vi "ThreePts_RotationMatrix.vi"(2 "Circumcenter":dbl[](array[numeric]), 3 "V 2":dbl[](array[numeric]), 4 "V 1":dbl[](array[numeric])) -> (0 "Circumcenter":dbl[](array[numeric]), 1 "Rotation Matrix ( Local to Global )":dbl[][](array[numeric]))   [LabVIEW 2016, in "ForceField.lvclass"]
uses:
  ForceField.lvclass
  <vilib>/Analysis/_algsub.llb/Real Vector Norm.vi
  <vilib>/Analysis/NI_AALPro.lvlib
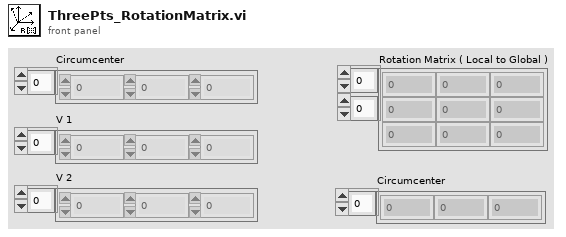
[diagram p1: front panel]
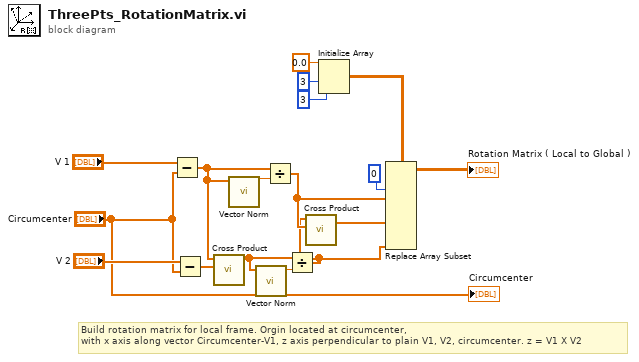
[diagram p0: block diagram]
diagram:
  # "Build rotation matrix for local frame. Orgin located at circumcenter, \nwith x axis along vector Circumcenter-V1, z axis perpendicular to plain V1, V2, circumcenter. z = V1 X V2"
  n1 = Subtract(x="V 1", y="Circumcenter") -> (x-y=w5:dbl[])
  n2 = Subtract(x="V 2", y="Circumcenter") -> (x-y=w10:dbl[])
  n3 = call <vilib>:"Cross Product.vi"("B Vector"=w10, "A Vector"=w5) -> ("Cross Product"=w2:dbl[])  [unwired: 8 in, 1 out]
  n4 = call-poly <vilib>:"Vector Norm.vi"("Input Vector"=w5) -> ("norm"=w6:dbl)  [unwired: 9 in, 1 out]
  n5 = call-poly <vilib>:"Vector Norm.vi"("Input Vector"=w2) -> ("norm"=w3:dbl)  [unwired: 9 in, 1 out]
  n6 = Divide(x=w5, y=w6) -> (x/y=w4:dbl[])
  n7 = Divide(x=w2, y=w3) -> (x/y=w1:dbl[])
  n8 = call <vilib>:"Cross Product.vi"("B Vector"=w4, "A Vector"=w1) -> ("Cross Product"=w11:dbl[])  [unwired: 8 in, 1 out]
  n9 = Initialize Array(0.0 ("element"), 3 ("dimension size"), 3 ("dimension size")) -> (w13:dbl[][])
  n10 = Replace Array Subset(array=w13, new element #1=w4, index (col) #1=0 ("disabled index (col)"), new element #2=w11, new element #3=w1) -> (→"Rotation Matrix ( Local to Global )":dbl[][])  [unwired: 5 in]
  "Circumcenter" <- "Circumcenter"
